vi "CheckButtoneTrue.vi"(10 "IN":bool) -> (2 "OUT":T1, 3 "OUT":bool)   [LabVIEW 2017, in "libVariable.lvlib" / "LibFunction.lvlib"]
uses:
  LibFunction.lvlib
  controls/stateModeDevice.ctl
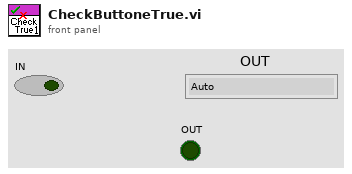
[diagram p1: front panel]
types:
  T1 = typedef "stateModeDevice.ctl" = enum16{"Auto", "Menu", "WaitAutoFinish", "Config", "initAuto"}
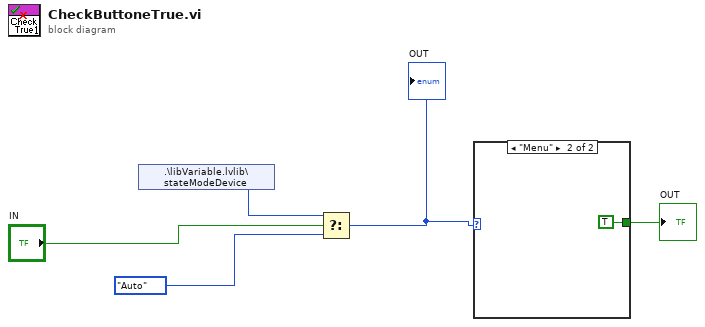
[diagram p0: block diagram]
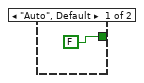
[diagram p2: hidden frame]
diagram:
  n1 = shared-variable ".\\libVariable.lvlib\\stateModeDevice"() -> (w5:T1)  [unwired: 1 in, 1 out]
  n2 = Select(t=w5, s="IN", f=stateModeDevice."Auto") -> (s? t:f=w2:T1)
  "OUT" <- w2
  n3 = case shown="\"Menu\"" w2 {
    tunnel: [FALSE ("OUT") TRUE ("OUT")] -> w1
    frame "Auto", Default {
    }
    frame "Menu" {
    }
  }
  "OUT" <- w1
